vi "4_1.vi"() -> ()   [LabVIEW 2015]
panel:
  out "Loop Counter":i32
  out "Match?":bool
  in  "stop":bool
  out "Current Number":u32
  in  "Number 2 Match":u32
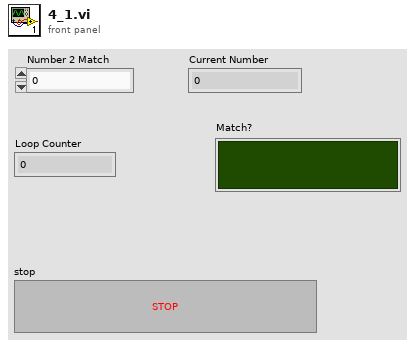
[diagram p1: front panel]
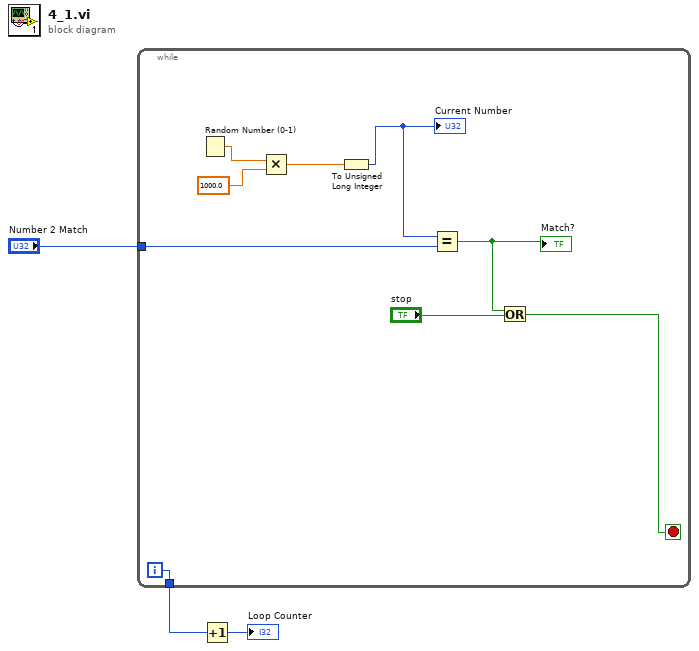
[diagram p0: block diagram]
diagram:
  n1 = while {
    tunnel: "Number 2 Match" -> [w9]
    tunnel: [w5] -> w2
    i -> [w5]
    stop <- w7 stop-if-true
    n2 = Random Number (0-1)() -> (number: 0 to 1=w4:dbl)
    n3 = Multiply(x=w4, y=1000.0) -> (x*y=w11:dbl)
    n4 = To Unsigned Long Integer(number=w11) -> (unsigned 32bit integer=w10:u32)
    "Current Number" <- w10
    n5 = Equal?(x=w10, y=w9) -> (x = y?=w6:bool)
    "Match?" <- w6
    n6 = Or(x=w6, y="stop") -> (x .or. y?=w7:bool)
  }
  n7 = Increment(x=w2) -> (x+1=→"Loop Counter":i32)
